vi "Read Artist.vi"(8 "error in (no error)":errorcluster, 11 "Song in":refnum<class "Song.lvclass">) -> (0 "error out":errorcluster, 2 "Artist":string, 3 "Song out":refnum<class "Song.lvclass">)   [LabVIEW 2015, in "Song.lvclass"]
uses:
  Song.lvclass
  Song.lvclass/Song.ctl
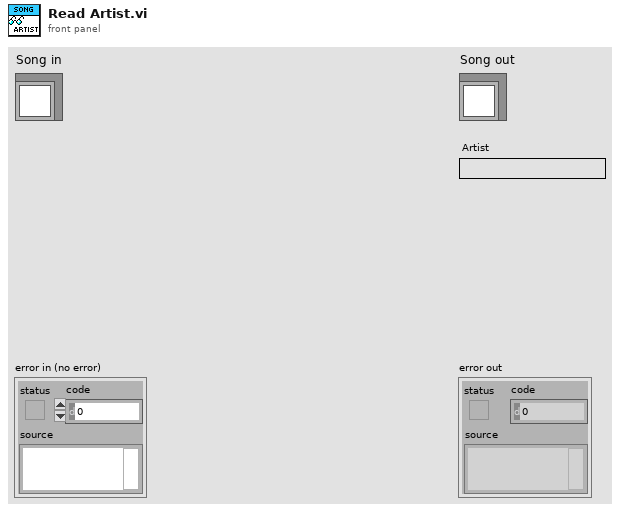
[diagram p1: front panel]
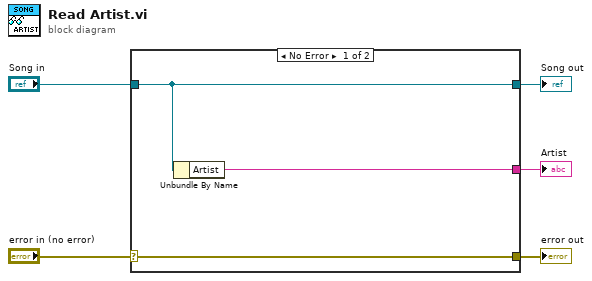
[diagram p0: block diagram]
diagram:
  n1 = case shown="No Error" "error in (no error)" {
    selector: "error in (no error)" -> [w8 w9]
    tunnel: [w8 w9] -> w4
    tunnel: [w7 w10] -> w2
    tunnel: "Song in" -> [w7 w10]
    tunnel: [w6 _] -> w1
    frame No Error {
      n2 = Unbundle By Name(w7) -> ("Artist"=w6:string)
    }
    frame Error {
    }
  }
  "error out" <- w4
  "Song out" <- w2
  "Artist" <- w1
